vi "A131258.vi"() -> ()   [LabVIEW 2020]
panel:
  out "零点标定":bool
  in  "工位滤波":cluster{"启用滤波":bool, "滤波系数":dbl}
  in  "右空载曲线":refnum<vi>
  in  "判定框参数":T1
  in  "结果判定参数":T2
  in  "坐标参数":T3
  in  "系数":T4
  in  "坐标参数":string[][](table)
  in  "右工位空载曲线":refnum<vi>
  in  "左工位空载曲线":refnum<vi>
  in  "最大压销力":dbl
  in  "右泄露":dbl
  in  "左泄露":dbl
  in  "逆向8":dbl
  in  "正向8":dbl
  in  "逆向5":dbl
  in  "正向5":dbl
  in  "逆向3":dbl
  in  "正向3":dbl
  in  "逆向1":dbl
  in  "正向1":dbl
  in  "对称性全":dbl
  in  "对称性5":dbl
  in  "对称性1":dbl
  in  "定点C":dbl
  in  "力位移曲线":refnum<vi>
  in  "LED-力位移":refnum<vi>
  in  "定点B":dbl
  in  "定点A":dbl
  in  "压力损失":cluster{"下限":dbl, "上限":dbl}
  in  "灵敏度":T5
  in  "内泄露曲线":refnum<vi>
  in  "压销力":cluster{"下限":dbl, "上限":dbl}
  in  "LED-自由间隙":refnum<vi>
  in  "LED-内泄露":refnum<vi>
  in  "LED-灵敏度":refnum<vi>
  in  "LED-磨合":refnum<vi>
  in  "内泄露":cluster{"下限":dbl, "上限":dbl}
  in  "试验项":enum32{"力特性", "压销位移力曲线"}(tab)
  in  "左空载曲线":refnum<vi>
  in  "自由间隙曲线":refnum<vi>
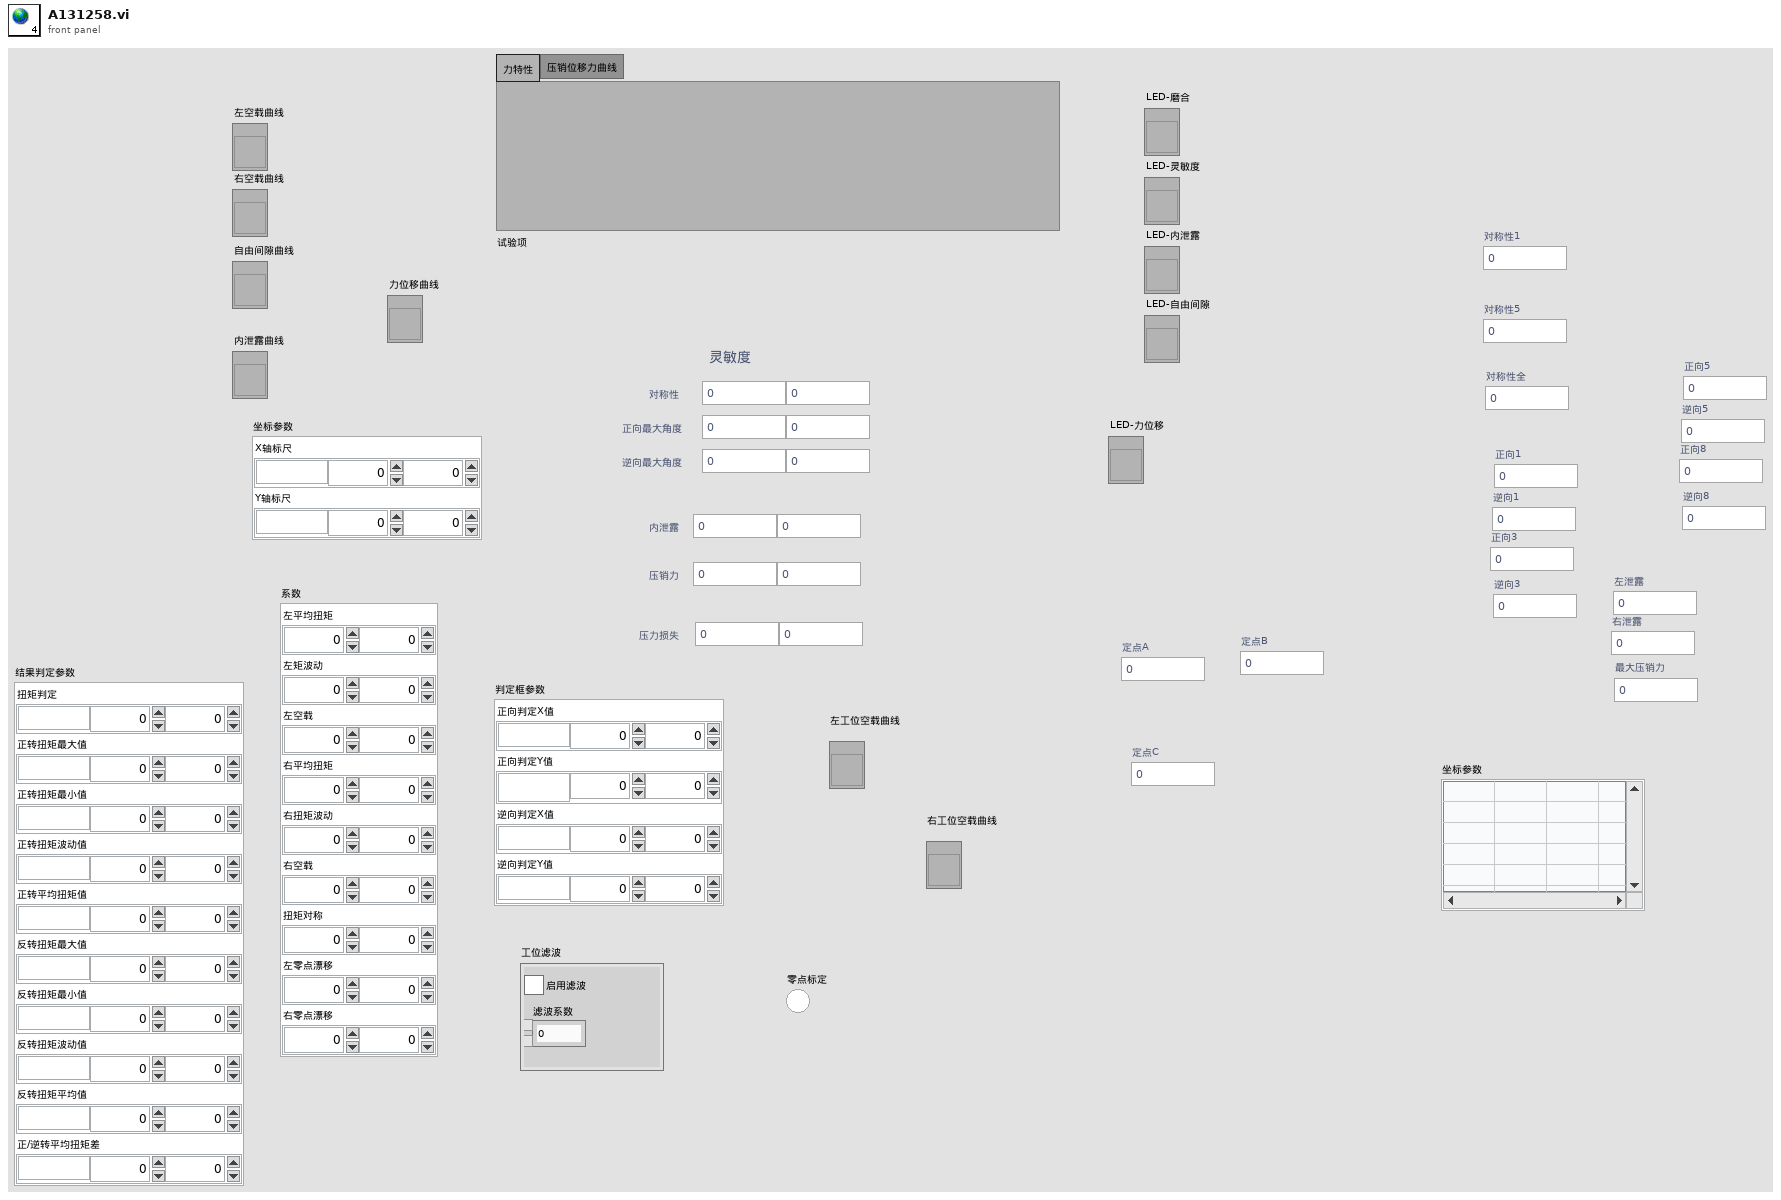
[diagram p1: front panel]
types:
  T1 = cluster{"正向判定X值":cluster{"单位":string, "下限":dbl, "上限":dbl}, "正向判定Y值":cluster{"单位":string, "下限":dbl, "上限":dbl}, "逆向判定X值":cluster{"单位":string, "下限":dbl, "上限":dbl}, "逆向判定Y值":cluster{"单位":string, "下限":dbl, "上限":dbl}}
  T2 = cluster{"扭矩判定":cluster{"单位":string, "下限":dbl, "上限":dbl}, "正转扭矩最大值":cluster{"单位":string, "下限":dbl, "上限":dbl}, "正转扭矩最小值":cluster{"单位":string, "下限":dbl, "上限":dbl}, "正转扭矩波动值":cluster{"单位":string, "下限":dbl, "上限":dbl}, "正转平均扭矩值":cluster{"单位":string, "下限":dbl, "上限":dbl}, "反转扭矩最大值":cluster{"单位":string, "下限":dbl, "上限":dbl}, "反转扭矩最小值":cluster{"单位":string, "下限":dbl, "上限":dbl}, "反转扭矩波动值":cluster{"单位":string, "下限":dbl, "上限":dbl}, "反转扭矩平均值":cluster{"单位":string, "下限":dbl, "上限":dbl}, "正/逆转平均扭矩差":cluster{"单位":string, "下限":dbl, "上限":dbl}}
  T3 = cluster{"X轴标尺":cluster{"单位":string, "下限":dbl, "上限":dbl}, "Y轴标尺":cluster{"单位":string, "下限":dbl, "上限":dbl}}
  T4 = cluster{"左平均扭矩":cluster{"正转":dbl, "反转":dbl}, "左矩波动":cluster{"正转":dbl, "反转":dbl}, "左空载":cluster{"正转":dbl, "反转":dbl}, "右平均扭矩":cluster{"正转":dbl, "反转":dbl}, "右扭矩波动":cluster{"正转":dbl, "反转":dbl}, "右空载":cluster{"正转":dbl, "反转":dbl}, "扭矩对称":cluster{"左":dbl, "右":dbl}, "左零点漂移":cluster{"正":dbl, "反":dbl}, "右零点漂移":cluster{"正":dbl, "反":dbl}}
  T5 = cluster{"         对称性":cluster{"下限":dbl, "上限":dbl}, "正向最大角度":cluster{"下限":dbl, "上限":dbl}, "逆向最大角度":cluster{"下限":dbl, "上限":dbl}}
diagram:
